vi "Set Result Settings.vi"(8 "error in (no error)":errorcluster, 10 "Analyze Parameter":refnum<class "Analyze Results Base.lvclass">, 11 "Analyze Fluence and Energy in":refnum<class "Analyze Fluence and Energy.lvclass">) -> (0 "error out":errorcluster, 3 "Analyze Fluence and Energy out":refnum<class "Analyze Fluence and Energy.lvclass">)   [LabVIEW 2014, in "Analyze.lvlib" / "Analyze Fluence and Energy.lvclass"]
uses:
  Analyze Fluence and Energy.lvclass
  Analyze Fluence/Analyze Fluence.lvclass
  Analyze Energy/Analyze Energy.lvclass
  Analyze Compound Analysis Base/Analyze Compound Analysis Base.lvclass
  Results and Overlays/Results Base/Analyze Results Base.lvclass
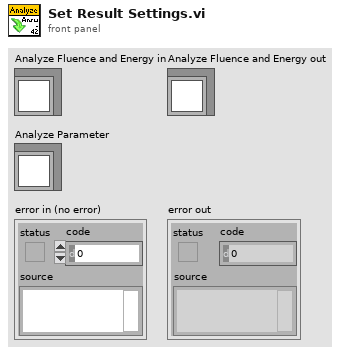
[diagram p1: front panel]
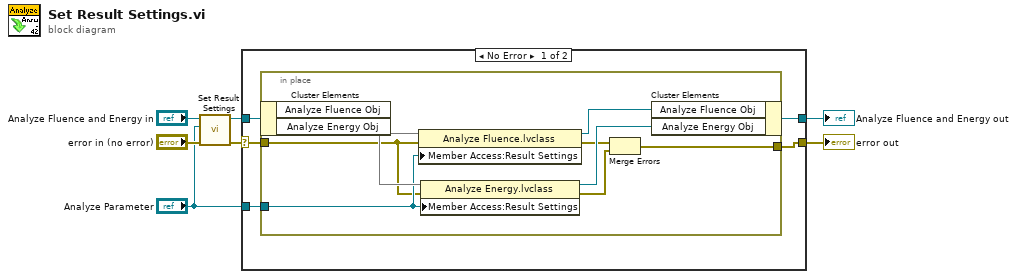
[diagram p0: block diagram]
diagram:
  n1 = call-parent "Set Result Settings.vi"("error in (no error)"="error in (no error)", "Analyze Parameter"="Analyze Parameter", "Analyze Compound Analysis Base in"="Analyze Fluence and Energy in") -> ("error out"=w4:errorcluster, "Analyze Compound Analysis Base out"=w5:refnum<class "Analyze Fluence and Energy.lvclass">)  [unwired: 7 in]
  n2 = case shown="No Error" w4 {
    selector: w4 -> [w11 w23]
    tunnel: [w9 w23] -> w2
    tunnel: [w10 w22] -> w3
    tunnel: w5 -> [w12 w22]
    tunnel: "Analyze Parameter" -> [w8 _]
    frame No Error {
      n3 = in-place {
        in-place-border: w11 -> [w16]
        in-place-border: w8 -> [w17]
        in-place-border: [w13] -> w9
        n4 = in-place-cluster #1(w12) -> ("Analyze Fluence Obj"=w21, "Analyze Energy Obj"=w20)
        n5 = property class="Analyze Fluence.lvclass"(reference=w21, error in=w16, "Member Access:Result Settings"=w17) -> (reference out=w18:refnum<class "Analyze Fluence.lvclass">, error out=w14:errorcluster)
        n6 = property class="Analyze Energy.lvclass"(reference=w20, error in=w16, "Member Access:Result Settings"=w17) -> (reference out=w19:refnum<class "Analyze Energy.lvclass">, error out=w15:errorcluster)
        n7 = Merge Errors(w14, w15) -> (w13:errorcluster)
        n8 = in-place-cluster #1("Analyze Fluence Obj"=w18, "Analyze Energy Obj"=w19) -> (w10:refnum<class "Analyze Fluence and Energy.lvclass">)
      }
    }
    frame Error {
    }
  }
  "error out" <- w2
  "Analyze Fluence and Energy out" <- w3
